vi "Check bytes at port.vi"(8 "error in (no error)":errorcluster, 11 "ArduinoAI in":refnum<class "ArduinoAI.lvclass">) -> (0 "error out":errorcluster, 1 "Bytes available":bool, 2 "Number of Bytes at Serial Port":u32, 3 "ArduinoAI out":refnum<class "ArduinoAI.lvclass">)   [LabVIEW 2020, in "ArduinoAI.lvclass"]
uses:
  ArduinoAI.lvclass
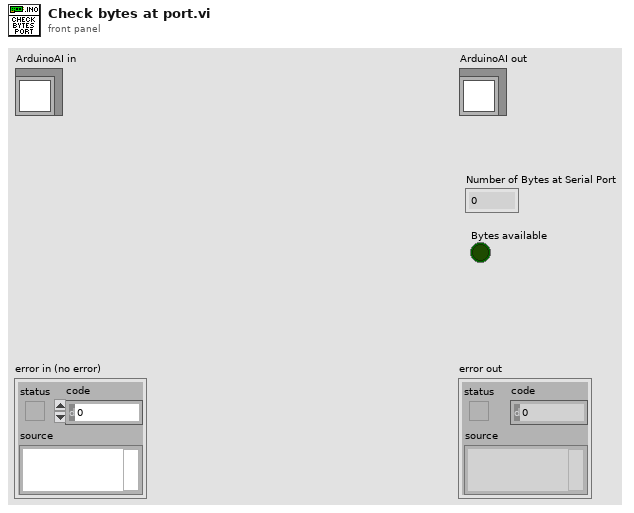
[diagram p1: front panel]
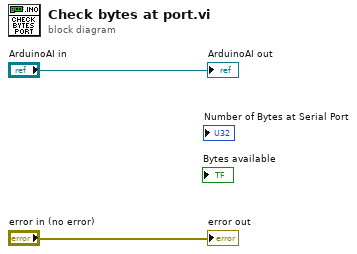
[diagram p0: block diagram]
diagram:
  "error out" <- "error in (no error)"
  "ArduinoAI out" <- "ArduinoAI in"
